vi "XY Plot - Label--Const.vi"() -> (3 "XY Plot Graph":string)   [LabVIEW 2017, in "DTacq Plot Display Library.lvlib"]
uses:
  DTacq Plot Display Library.lvlib
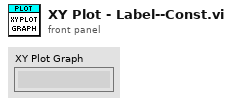
[diagram p1: front panel]
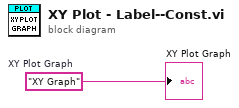
[diagram p0: block diagram]
diagram:
  w1 = "XY Graph"  # XY Plot Graph
  "XY Plot Graph" <- w1
